vi "Main.vi"(11 "Module Admin":refnum<class "Delacor_lib_QMH_Module Admin.lvclass">) -> ()   [LabVIEW 2019, in "FileReader.lvlib"]
doc: "This template is based off of the Queued Message Handler design pattern and the Queued Message Handler project template that ships with LabVIEW.\n\nThe main difference is that the queue is private to this module and communication between modules is performed via Broadcast and Request events.\n\nRequest events are wrapped in public API methods and are handled in the Event Handling Loop (EHL) of this VI. Any module can register for Broadcast events sent by this module. The EHL generates messages based on user interface actions.\n\nThe Message Handling Loop (MHL) processes messages generated by the EHL, or by other messages. The messages are string values, so new messages can be added easily to the Message Cases case structure in the MHL. Each message cluster can also provide an optional value for Message Data, which is a variant that can be converted to whatever message-specific data is required.\n_____\nBased on Delacor QMH Project Template 4.0.0.47.\n_____\nBased on DQMH Project Template 6.1.0.94."
uses:
  FileReader.lvlib
  <vilib>/Delacor/Delacor QMH/Libraries/Module Admin_class/Delacor_lib_QMH_Module Admin.lvclass
  Neo-Laura-LVOOP/SignalViewer/TDMS_DataHandler_class/TDMS_DataHandler.lvclass
  Stop Argument--cluster.ctl
  <vilib>/Delacor/Delacor QMH/Libraries/Message Queue_class/Delacor_lib_QMH_Message Queue.lvclass/Delacor_lib_QMH_Message Queue.ctl
  <vilib>/Delacor/Delacor QMH/Libraries/Module Admin_class/Delacor_lib_QMH_Module Admin.lvclass/Delacor_lib_QMH_Module Admin.ctl
  Open TDMS file Argument--cluster.ctl
  Open TDMS file (Reply Payload)--cluster.ctl
  Neo-Laura-LVOOP/SignalViewer/TDMS_DataHandler_class/Fcurve Meta data.ctl
  Filepath Editor/Update Application Settings (Reply Payload)--cluster.ctl
  Filepath Editor/Settings--cluster.ctl
  <vilib>/Utility/miscctls.llb/LVPointTypeDef.ctl
  <vilib>/Delacor/Delacor QMH/Libraries/Message Queue_class/Delacor_lib_QMH_Enqueue Message (Single).vi
  <vilib>/Delacor/Delacor QMH/Libraries/Module Admin_class/Delacor_lib_QMH_Get External Launch.vi
  <vilib>/Utility/error.llb/Error Cluster From Error Code.vi
  <vilib>/ErrorRing/Error Ring.xnode
  <vilib>/Delacor/Delacor QMH/Libraries/Message Queue_class/Delacor_lib_QMH_Message Queue.lvclass
  Filepath Editor/Filepath Editor.lvlib
panel:
  out "error out":errorcluster
  # "This is a headless module. Show its panel to confirm that the Settings are updated correctly and other debugging tasks. Use the Settings Editor to change the settings for this module."
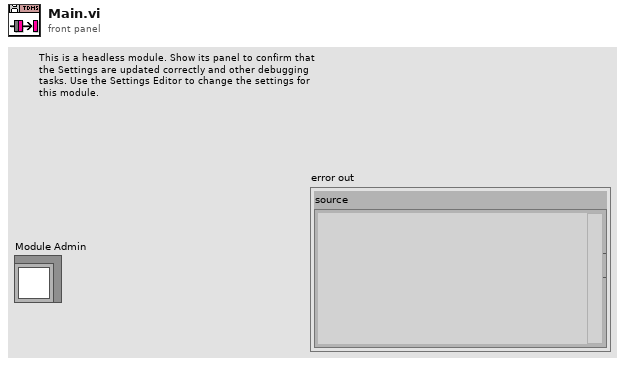
[diagram p1: front panel]
types:
  T1 = typedef "Filepath Editor.lvlib/Broadcast Events--cluster.ctl" = cluster{"Module Did Init":refnum<user-event>, "Status Updated":refnum<user-event>, "Error Reported":refnum<user-event>, "Module Did Stop":refnum<user-event>, "Update Module Execution Status":refnum<user-event>, "TDMS path settings updated":refnum<user-event>}
  T2 = typedef "FileReader.lvlib/Request Events--cluster.ctl" = cluster{"Stop Module":refnum<user-event>, "Show Panel":refnum<user-event>, "Hide Panel":refnum<user-event>, "Get Module Execution Status":refnum<user-event>, "Show Diagram":refnum<user-event>, "Open TDMS file":refnum<user-event>}
  T3 = enum32{"invalid lock state", "Not Locked", "Locked (No Password)", "Password-protected"}
  T4 = typedef "FileReader.lvlib/Stop Argument--cluster.ctl" = cluster{"Origin":string, "Exit via Stop Module Req?":bool, "Wait for Module to stop?":bool}
  T5 = typedef "FileReader.lvlib/Open TDMS file Argument--cluster.ctl" = cluster{"Wait Notifier":refnum<notifier>, "wait for reply":bool, "TDMS filepath":path}
  T6 = typedef "Update Application Settings (Reply Payload)--cluster.ctl" = cluster{"Settings":T7, "error":errorcluster}
  T7 = typedef "Filepath Editor.lvlib/Settings--cluster.ctl" = cluster{"TDMS Filepath":path, "TDMS Directory":path, "Dir?":bool}
  T8 = typedef "LVPointTypeDef.ctl" = cluster{"Horizontal":i16, "Vertical":i16}
  T9 = enum32{"Invalid", "Standard", "Closed", "Hidden", "Minimized", "Maximized"}
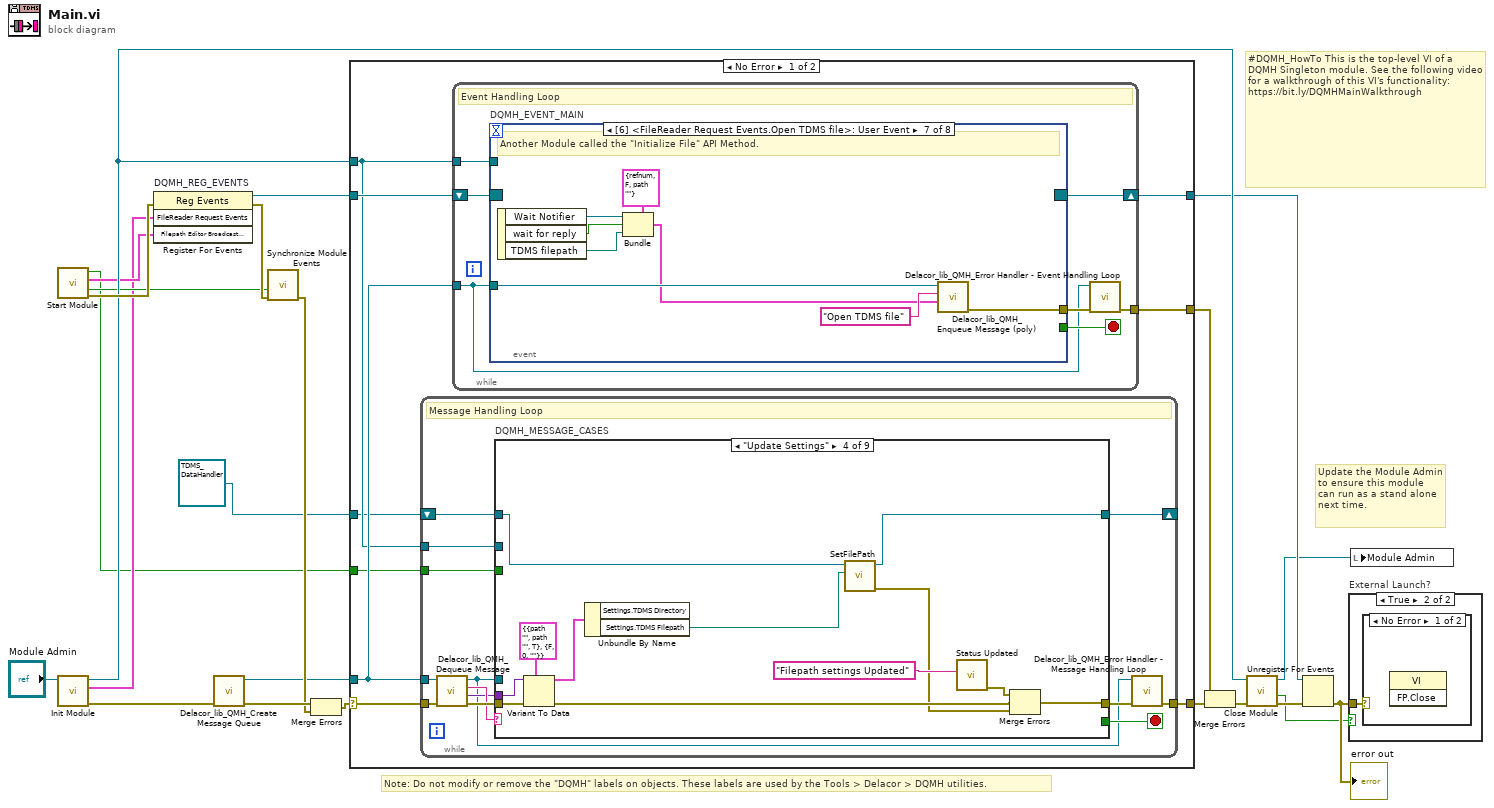
[diagram p0: block diagram]
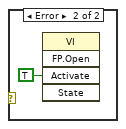
[diagram p3: hidden frame]
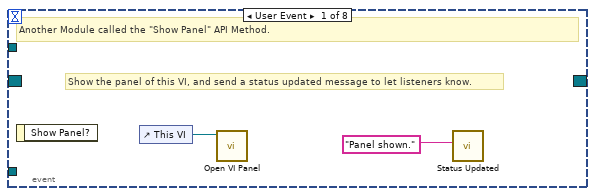
[diagram p4: hidden frame]
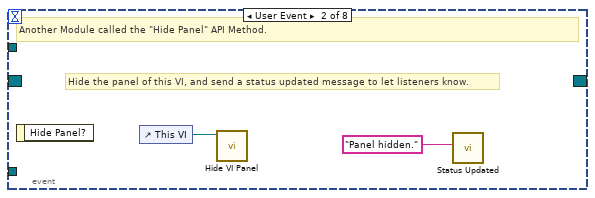
[diagram p5: hidden frame]
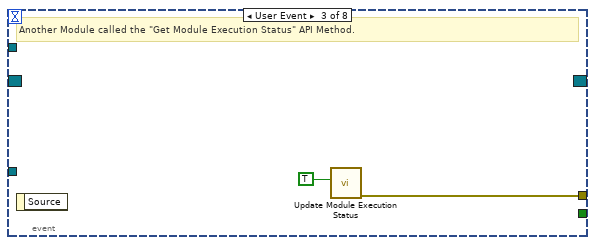
[diagram p6: hidden frame]
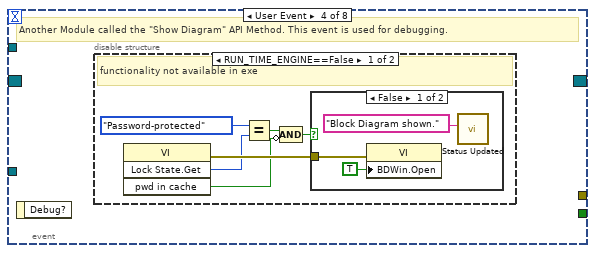
[diagram p7: hidden frame]
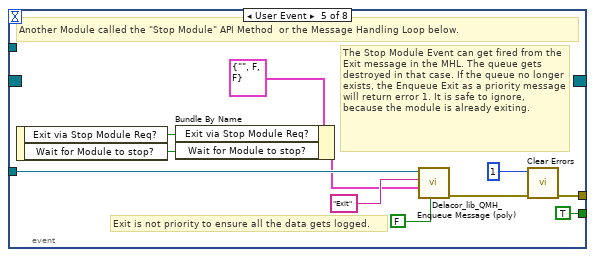
[diagram p10: hidden frame]
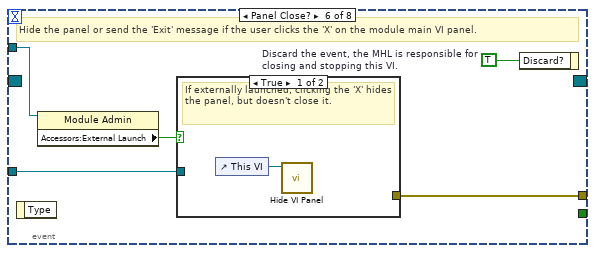
[diagram p11: hidden frame]
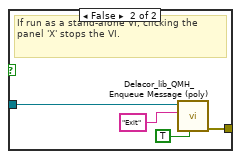
[diagram p12: hidden frame]
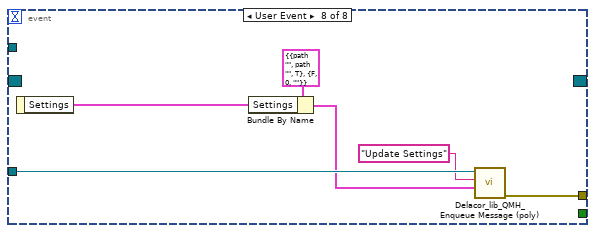
[diagram p13: hidden frame]
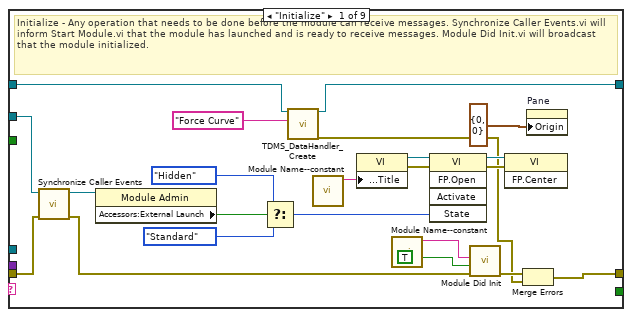
[diagram p14: hidden frame]
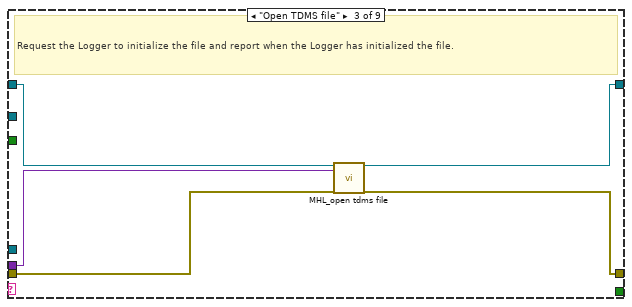
[diagram p16: hidden frame]
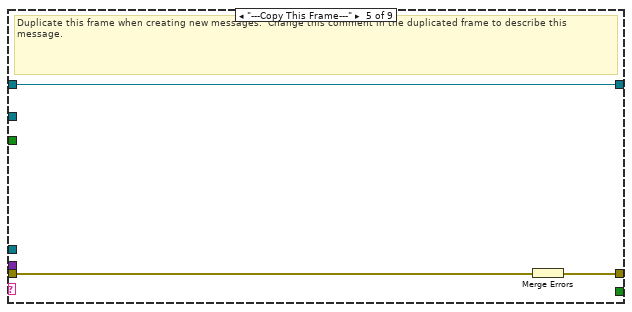
[diagram p17: hidden frame]
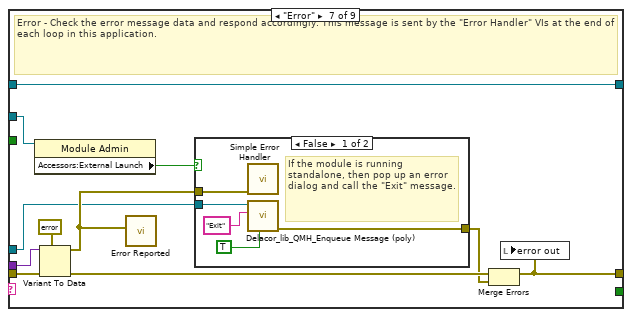
[diagram p19: hidden frame]
diagram:
  # "#DQMH_HowTo This is the top-level VI of a DQMH Singleton module. See the following video for a walkthrough of this VI's functionality: https://bit.ly/DQMHMainWalkthrough"
  # "Note: Do not modify or remove the \"DQMH\" labels on objects. These labels are used by the Tools > Delacor > DQMH utilities."
  # "Update the Module Admin to ensure this module can run as a stand alone next time."
  n1 = call "Start Module.vi"() -> ("error out"=w15:errorcluster, "Wait for Event Sync?"=w5:bool, "Filepath Editor Broadcast Events"=w4:T1, "Module Was Already Running?"=w2:bool)  [unwired: 8 in]
  n2 = call "Init Module.vi"("Singleton Module Admin in"="Module Admin") -> ("error out"=w22:errorcluster, "FileReader Request Events"=w3:T2, "Singleton Module Admin out"=w12:refnum<class "Delacor_lib_QMH_Module Admin.lvclass">)  [unwired: 8 in]
  n3 = register-events "DQMH_REG_EVENTS"(error in=w15, w3, w4) -> (reference out=w10:refnum<event-registration>, error out=w14:errorcluster)  [unwired: 1 in]
  n4 = call <vilib>:"Delacor_lib_QMH_Create Message Queue.vi"("error in"=w22) -> ("error out"=w17:errorcluster, "Message Queue"=w9:refnum<class "Delacor_lib_QMH_Message Queue.lvclass">)  [unwired: 9 in]
  n5 = call "Synchronize Module Events.vi"("error in (no error)"=w14, "Wait for Event Sync?"=w5) -> ("error out"=w13:errorcluster)  [unwired: 9 in]
  n6 = Merge Errors(w17, w13) -> (w16:errorcluster)
  n7 = case shown="No Error" w16 {
    selector: w16 -> [w30 w200]
    tunnel: [w32 w199] -> w23
    tunnel: [w29 w207] -> w11
    tunnel: w10 -> [w28 w207]
    tunnel: w9 -> [w27 w201]
    tunnel: [w31 _] -> w20
    tunnel: w12 -> [w26 w203]
    tunnel: w2 -> [w25 w202]
    tunnel: refnum<class "TDMS_DataHandler.lvclass"> refnum ("DataHandler") -> [w24 _]
    frame No Error {
      n8 = while {
        tunnel: w27 -> [w93]
        shift-right: [w97] -> _
        shift-left: w24 -> [w98]
        tunnel: w30 -> [w101]
        tunnel: [w99] -> w32
        tunnel: w26 -> [w91]
        tunnel: w25 -> [w90]
        stop <- w96 stop-if-true
        # "Message Handling Loop"
        n9 = call-dynamic "Delacor_lib_QMH_Dequeue Message.vi"("error in"=w101, "Message Queue in"=w93) -> ("error out"=w100:errorcluster, "Message Data"=w94:variant, "Message"=w95:string, "Message Queue out"=w92:refnum<class "Delacor_lib_QMH_Message Queue.lvclass">)  [unwired: 6 in]
        n10 = case "DQMH_MESSAGE_CASES" shown="\"Update Settings\"" w95 {
          selector: w95 -> [_ _ _ _ _ _ _ _ w186]
          tunnel: w92 -> [_ _ _ _ _ _ w151 w176 _]
          tunnel: w100 -> [w122 w126 w131 w143 w146 w148 w158 w182 w188]
          tunnel: [w119 w126 w127 w134 w145 w148 w154 w179 w189] -> w102
          tunnel: w98 -> [w104 w125 w128 w137 w144 w147 w153 w167 w187]
          tunnel: [w105 w125 w129 w136 w144 w147 w153 w165 w187] -> w97
          tunnel: [_ _ _ _ _ _ _ w175 _] -> w96
          tunnel: w94 -> [_ _ w130 w142 _ _ w152 w174 _]
          tunnel: w91 -> [w111 _ _ _ _ _ w150 w169 _]
          tunnel: w90 -> [_ _ _ _ _ _ _ w168 _]
          frame "Initialize" {
            # "Initialize - Any operation that needs to be done before the module can receive messages. Synchronize Caller Events.vi will inform Start Module.vi that the module has launched and is ready to receive messages. Module Did Init.vi will broadcast that the module initialized."
            n11 = call "Synchronize Caller Events.vi"("error in (no error)"=w122, "Singleton Module Admin in"=w111) -> ("error out"=w121:errorcluster, "Singleton Module Admin out"=w108:refnum<class "Delacor_lib_QMH_Module Admin.lvclass">)  [unwired: 8 in]
            n12 = property class="Module Admin"(reference=w108) -> ("Accessors:External Launch"=w115:bool)  [unwired: 1 in, 2 out]
            n13 = Select(t=T9."Hidden" ("State"), s=w115, f=T9."Standard" ("State")) -> (s? t:f=w112:T9)
            n14 = call "TDMS_DataHandler_Create.vi"("reference in"=w104, "Group name"="Force Curve") -> ("reference out"=w105:refnum<class "TDMS_DataHandler.lvclass">, "error out"=w103:errorcluster)  [unwired: 16 in]
            n15 = call "Module Name--constant.vi"() -> ("Module Name"=w118:string)  [unwired: 11 in]
            n16 = property class="VI"("Front Panel.Title"=w118) -> (reference out=w117:refnum<vi>, error out=w124:errorcluster)  [unwired: 2 in]
            n17 = call "Module Name--constant.vi"() -> ("Module Name"=w109:string)  [unwired: 11 in]
            n18 = invoke class="VI" method="FP.Open"(reference=w117, error in=w124, "State"=w112) -> (reference out=w116:refnum<vi>, error out=w123:errorcluster)  [unwired: 2 in, 3 out]
            n19 = call "Module Did Init.vi"("error in (no error)"=w121, "Initialized?"=TRUE, "Origin"=w109) -> ("error out"=w120:errorcluster)  [unwired: 8 in]
            n20 = invoke class="VI" method="FP.Center"(reference=w116, error in=w123) -> ()  [unwired: 1 in, 3 out]
            n21 = Merge Errors(w120, w103) -> (w119:errorcluster)
            n22 = property on="Pane" class="Pane"("Origin"=T8 {"Horizontal"=0, "Vertical"=0}) -> ()  [unwired: 2 in, 2 out]
          }
          frame "---Module Specific---" {
            # "Separator -- The following cases handle messages specific to this Module."
          }
          frame "Open TDMS file" {
            # "Request the Logger to initialize the file and report when the Logger has initialized the file."
            n23 = call "MHL_open tdms file.vi"("TDMS_DataHandler in"=w128, "Message Data"=w130, "error in (no error)"=w131) -> ("TDMS_DataHandler out"=w129:refnum<class "TDMS_DataHandler.lvclass">, "error out"=w127:errorcluster)  [unwired: 15 in]
          }
          frame "Update Settings" {
            n24 = Variant To Data(error in=w143, type=T6 {"Settings"={"TDMS Filepath"=path "", "TDMS Directory"=path "", "Dir?"=TRUE}, "error"={"status"=FALSE, "code"=0, "source"=""}} ("Settings Updated Argument"), Variant=w142) -> (data=w141:T6, error out=w135:errorcluster)
            n25 = Unbundle By Name(w141) -> ("Settings.TDMS Filepath"=w138:path)  [unwired: 1 out]
            n26 = call-dynamic "SetFilePath.vi"("Filepath"=w138, "reference in"=w137) -> ("error out"=w133:errorcluster, "reference out"=w136:refnum<class "TDMS_DataHandler.lvclass">)  [unwired: 8 in]
            n27 = call "Status Updated.vi"("Status"="Filepath settings Updated") -> ("error out"=w132:errorcluster)  [unwired: 10 in]
            n28 = Merge Errors(w132, w135, w133) -> (w134:errorcluster)
          }
          frame "---Copy This Frame---" {
            # "Duplicate this frame when creating new messages.  Change this comment in the duplicated frame to describe this message."
            n29 = Merge Errors(w146) -> (w145:errorcluster)
          }
          frame "---Exit and Error Handling---" {
            # "Separator - The following cases handle errors and exit messages."
          }
          frame "Error" {
            # "Error - Check the error message data and respond accordingly. This message is sent by the \"Error Handler\" VIs at the end of each loop in this application."
            n30 = property class="Module Admin"(reference=w150) -> ("Accessors:External Launch"=w149:bool)  [unwired: 1 in, 2 out]
            n31 = Variant To Data(error in=w158, type=errorcluster {"status"=FALSE, "code"=0, "source"=""} ("error constant"), Variant=w152) -> (data=w159:errorcluster, error out=w156:errorcluster)
            n32 = call "Error Reported.vi"("Error"=w159) -> ()  [unwired: 10 in, 1 out]
            n33 = case shown="False" w149 {
              tunnel: [w164 _] -> w155
              tunnel: w151 -> [w162 _]
              tunnel: w159 -> [w163 _]
              frame False {
                # "If the module is running standalone, then pop up an error dialog and call the \"Exit\" message."
                n34 = call <vilib>:"Simple Error Handler.vi"("error in (no error)"=w163) -> ()  [unwired: 4 in, 5 out]
                n35 = call-poly <vilib>:"Delacor_lib_QMH_Enqueue Message (poly).vi"("Priority Message? (F)"=TRUE, "Message"="Exit", "Message Queue in"=w162) -> ("error out"=w164:errorcluster)  [unwired: 7 in, 1 out]
              }
              frame True {
                # "If the module was launched externally, calling the Error Reported broadcast VI is the only action performed by the \"Error\" message. The module's caller can then process the error appropriately."
              }
            }
            n36 = Merge Errors(w156, w155) -> (w154:errorcluster)
            n37 = local write "error out"(w154) -> ()
          }
          frame "Exit" {
            w173 = 91  # 91: not all Exit messages will have an argument
            w175 = TRUE  # Stop the VI
            # "Release the message queue reference"
            # "Exit - Exit the application."
            n38 = Variant To Data(error in=w182, type=T4 {"Origin"="", "Exit via Stop Module Req?"=FALSE, "Wait for Module to stop?"=FALSE} ("Stop Argument"), Variant=w174) -> (data=w171:T4, error out=w178:errorcluster)
            n39 = call <vilib>:"Clear Errors.vi"("error in (no error)"=w178, "specific error code to clear (0: all)"=w173) -> ("error out"=w181:errorcluster)  [unwired: 4 in, 1 out]
            n40 = control-ref of="This VI"() -> (w170:refnum<vi>)
            n41 = call-dynamic "Delacor_lib_QMH_Release Message Queue.vi"("error in"=w181, "Message Queue"=w176) -> ("error out"=w180:errorcluster)  [unwired: 9 in]
            n42 = call "Handle Exit.vi"("Stop Argument"=w171, "Admin in"=w169, "VI reference"=w170) -> ("error out"=w177:errorcluster)  [unwired: 7 in, 1 out]
            n43 = call-dynamic "Destroy.vi"("reference in"=w167) -> ("reference out"=w165:refnum<class "TDMS_DataHandler.lvclass">, "error out"=w166:errorcluster)  [unwired: 17 in]
            n44 = case "Settings Editor was\nalready running?" shown="False" w168 {
              frame False {
                n45 = call "Module Name--constant.vi"() -> ("Module Name"=w184:string)  [unwired: 11 in]
                n46 = call "Stop Module.vi"("Wait for Module to Stop? (F)"=TRUE, "Origin"=w184) -> ()  [unwired: 9 in, 1 out]
              }
              frame True {
                # "Another Module is\nin charge of stopping Settings Editor"
              }
            }
            n47 = Merge Errors(w166, w180, w177) -> (w179:errorcluster)
          }
          frame Default {
            # "'Default' case only runs if there is a message that isn't defined in any of the other cases.  Output a programming error."
            n48 = call "Module Name--constant.vi"() -> ("Module Name"=w185:string)  [unwired: 11 in]
            n49 = xnode "Error Ring"("parameter 0"=w186, "parameter 1"=w185) -> ("error out"=w190:errorcluster)
            n50 = Merge Errors(w188, w190) -> (w189:errorcluster)
          }
        }
        n51 = call-dynamic "Delacor_lib_QMH_Error Handler - Message Handling Loop.vi"("error in"=w102, "Message Queue in"=w92) -> ("dup error in"=w99:errorcluster)  [unwired: 8 in, 1 out]
      }
      n52 = while {
        tunnel: w27 -> [w33]
        shift-right: [w36] -> w29
        shift-left: w28 -> [w37]
        tunnel: [w38] -> w31
        tunnel: w26 -> [w34]
        stop <- w35 stop-if-true
        # "Event Handling Loop"
        n53 = event "DQMH_EVENT_MAIN" shown="[6] <FileReader Request Events.Open TDMS file>: User Event" {
          selector: w37 -> [_ _ _ _ _ _ _ _]
          dyn-events: [_ _ _ _ _ _ _ _] -> w36
          timeout: _ -> [_ _ _ _ _ _ _ _]
          tunnel: [_ _ _ _ TRUE ("Discard?") _ _ _] -> w35
          tunnel: w33 -> [_ _ _ _ w61 w68 w82 w88]
          tunnel: [_ _ w45 _ w64 w70 w83 w89] -> w39
          tunnel: w34 -> [_ _ _ _ _ w67 _ _]
          event User Event {
            # "Show the panel of this VI, and send a status updated message to let listeners know."
            # "Another Module called the \"Show Panel\" API Method."
            n54 = event-data() -> ()  [unwired: 1 in, 1 out]
            n55 = control-ref of="This VI"() -> (w41:refnum<vi>)
            n56 = call "Open VI Panel.vi"("VI"=w41) -> ()  [unwired: 10 in, 1 out]
            n57 = call "Status Updated.vi"("Status"="Panel shown." ("format string")) -> ()  [unwired: 10 in, 1 out]
          }
          event User Event {
            # "Hide the panel of this VI, and send a status updated message to let listeners know."
            # "Another Module called the \"Hide Panel\" API Method."
            n58 = event-data() -> ()  [unwired: 1 in, 1 out]
            n59 = control-ref of="This VI"() -> (w43:refnum<vi>)
            n60 = call "Hide VI Panel.vi"("VI"=w43) -> ()  [unwired: 10 in, 1 out]
            n61 = call "Status Updated.vi"("Status"="Panel hidden." ("format string")) -> ()  [unwired: 10 in, 1 out]
          }
          event User Event {
            # "Another Module called the \"Get Module Execution Status\" API Method."
            n62 = event-data() -> ()  [unwired: 1 in, 1 out]
            n63 = call "Update Module Execution Status.vi"("Running?"=TRUE) -> ("error out"=w45:errorcluster)  [unwired: 10 in]
          }
          event User Event {
            # "Another Module called the \"Show Diagram\" API Method. This event is used for debugging."
            n64 = event-data() -> ()  [unwired: 1 in, 1 out]
            n65 = disable-structure shown="RUN_TIME_ENGINE==False" {
              frame condition #0 (active) {
                # "functionality not available in exe"
                n66 = invoke class="VI" method="Lock State.Get"() -> (error out=w51:errorcluster, "Get Lock State"=w50:T3, "pwd in cache"=w47:bool)  [unwired: 4 in, 1 out]
                n67 = Equal?(x=T3."Password-protected", y=w50) -> (x = y?=w48:bool)
                n68 = Compound Arithmetic op=AND(w48, invert w47) -> (w46:bool)
                n69 = case shown="False" w46 {
                  tunnel: w51 -> [w54 _]
                  frame False {
                    n70 = property class="VI"(error in=w54, "BDWin.Open"=TRUE ("Block Diagram Window:Open")) -> ()  [unwired: 1 in, 2 out]
                    n71 = call "Status Updated.vi"("Status"="Block Diagram shown." ("format string")) -> ()  [unwired: 10 in, 1 out]
                  }
                  frame True {
                    # "Password-protected VI, and the password is not in the cache. Do not show the diagram."
                  }
                }
              }
              frame condition #1 {
              }
            }
          }
          event User Event {
            # "Exit is not priority to ensure all the data gets logged."
            # "The Stop Module Event can get fired from the Exit message in the MHL. The queue gets destroyed in that case. If the queue no longer exists, the Enqueue Exit as a priority message will return error 1. It is safe to ignore, because the module is already exiting."
            # "Another Module called the \"Stop Module\" API Method  or the Message Handling Loop below."
            n72 = event-data() -> ("Exit via Stop Module Req?"=w57:bool, "Wait for Module to stop?"=w56:bool)  [unwired: 1 in]
            n73 = Bundle By Name(cluster=T4 {"Origin"="", "Exit via Stop Module Req?"=FALSE, "Wait for Module to stop?"=FALSE} ("Stop Argument"), "Exit via Stop Module Req?"=w57, "Wait for Module to stop?"=w56) -> (w55:T4)
            n74 = call-poly <vilib>:"Delacor_lib_QMH_Enqueue Message (poly).vi"("Priority Message? (F)"=FALSE, "Message Data"=w55, "Message"="Exit", "Message Queue in"=w61) -> ("error out"=w65:errorcluster)  [unwired: 6 in, 1 out]
            n75 = call <vilib>:"Clear Errors.vi"("error in (no error)"=w65, "specific error code to clear (0: all)"=1) -> ("error out"=w64:errorcluster)  [unwired: 4 in, 1 out]
          }
          event Panel Close? {
            w69 = TRUE  # Discard the event, the MHL is responsible for closing and stopping this VI.
            # "Hide the panel or send the 'Exit' message if the user clicks the 'X' on the module main VI panel."
            n76 = event-data() -> ()  [unwired: 1 in, 1 out]
            n77 = property class="Module Admin"(reference=w67) -> ("Accessors:External Launch"=w66:bool)  [unwired: 1 in, 2 out]
            n78 = case shown="True" w66 {
              tunnel: w68 -> [_ w74]
              tunnel: [_ w75] -> w70
              frame True {
                # "If externally launched, clicking the 'X' hides the panel, but doesn't close it."
                n79 = control-ref of="This VI"() -> (w71:refnum<vi>)
                n80 = call "Hide VI Panel.vi"("VI"=w71) -> ()  [unwired: 10 in, 1 out]
              }
              frame False {
                # "If run as a stand-alone VI, clicking the panel 'X' stops the VI."
                n81 = call-poly <vilib>:"Delacor_lib_QMH_Enqueue Message (poly).vi"("Priority Message? (F)"=TRUE, "Message"="Exit", "Message Queue in"=w74) -> ("error out"=w75:errorcluster)  [unwired: 7 in, 1 out]
              }
            }
            n82 = event-data("Discard?"=w69) -> ()  [unwired: 1 in, 1 out]
          }
          event User Event {
            # "Another Module called the \"Initialize File\" API Method."
            n83 = event-data() -> ("Wait Notifier"=w78:refnum<notifier>, "wait for reply"=w77:bool, "TDMS filepath"=w76:path)  [unwired: 1 in]
            n84 = Bundle(cluster=T5 {"Wait Notifier"=refnum, "wait for reply"=FALSE, "TDMS filepath"=path ""} ("Initialize File Argument"), "Wait Notifier"=w78, "wait for reply"=w77, "TDMS filepath"=w76) -> (w79:T5)
            n85 = call-poly <vilib>:"Delacor_lib_QMH_Enqueue Message (poly).vi"("Message Data"=w79, "Message"="Open TDMS file", "Message Queue in"=w82) -> ("error out"=w83:errorcluster)  [unwired: 7 in, 1 out]
          }
          event User Event {
            n86 = event-data() -> ("Settings"=w85:T7)  [unwired: 1 in]
            n87 = Bundle By Name(cluster=T6 {"Settings"={"TDMS Filepath"=path "", "TDMS Directory"=path "", "Dir?"=TRUE}, "error"={"status"=FALSE, "code"=0, "source"=""}} ("Settings Updated Argument"), "Settings"=w85) -> (w84:T6)
            n88 = call-poly <vilib>:"Delacor_lib_QMH_Enqueue Message (poly).vi"("Message Data"=w84, "Message"="Update Settings", "Message Queue in"=w88) -> ("error out"=w89:errorcluster)  [unwired: 7 in, 1 out]
          }
        }
        n89 = call-dynamic "Delacor_lib_QMH_Error Handler - Event Handling Loop.vi"("error in"=w39, "Message Queue in"=w33) -> ("dup error in"=w38:errorcluster)  [unwired: 8 in, 1 out]
      }
    }
    frame Error {
      # "Synchronize Caller Events.vi will inform Start Module.vi that the module has launched and will let the code calling Start Module.vi register for broadcasts and would permit the caller receive the broadcast that an error occurred at launch time."
      n90 = call "Synchronize Caller Events.vi"("Singleton Module Admin in"=w203) -> ("error out"=w208:errorcluster)  [unwired: 9 in, 1 out]
      n91 = call-dynamic "Delacor_lib_QMH_Release Message Queue.vi"("error in"=w200, "Message Queue"=w201) -> ("error out"=w199:errorcluster)  [unwired: 9 in]
      n92 = call "Module Name--constant.vi"() -> ("Module Name"=w206:string)  [unwired: 11 in]
      n93 = case "Settings Editor was\nalready running?" shown="False" w202 {
        frame False {
          n94 = call "Module Name--constant.vi"() -> ("Module Name"=w211:string)  [unwired: 11 in]
          n95 = call "Stop Module.vi"("Wait for Module to Stop? (F)"=TRUE, "Origin"=w211) -> ()  [unwired: 9 in, 1 out]
        }
        frame True {
          # "Another Module is\nin charge of stopping Settings Editor"
        }
      }
      n96 = Format Into String(format string="An error occurred during initialization. %s is no longer running.", w206) -> (resulting string=w204:string)  [unwired: 2 in, 1 out]
      n97 = Merge Errors(w200, w208) -> (w209:errorcluster)
      n98 = call "Error Reported.vi"("Additional Information"=w204, "Error"=w209) -> ()  [unwired: 9 in, 1 out]
    }
  }
  n99 = Merge Errors(w20, w23) -> (w19:errorcluster)
  n100 = call "Close Module.vi"("error in (no error)"=w19, "Module Admin in"=w12) -> ("error out"=w21:errorcluster, "External Launch"=w6:bool, "Module Admin out"=w7:refnum<class "Delacor_lib_QMH_Module Admin.lvclass">)  [unwired: 7 in]
  n101 = Unregister For Events(event registration refnum=w11, error in=w21) -> (error out=w18:errorcluster)
  "error out" <- w18
  n102 = case "External Launch?" shown="True" w6 {
    tunnel: w18 -> [_ w212]
    frame False {
    }
    frame True {
      n103 = case shown="No Error" w212 {
        frame No Error {
          n104 = invoke class="VI" method="FP.Close"() -> ()  [unwired: 3 in, 3 out]
        }
        frame Error {
          n105 = invoke class="VI" method="FP.Open"("Activate"=TRUE ("Activate?")) -> ()  [unwired: 4 in, 5 out]
        }
      }
    }
  }
  n106 = local write "Module Admin"(w7) -> ()
